vi "KE622x -- Set Arm Layer Params.vi"(0 "Resource In":refnum<visa-resource-name>, 1 "Check For SCPI Errors? (T)":bool=TRUE, 7 "Arm Layer Params In":T1={"Bypass Arm Layer\nInput Trigger?"=FALSE, "Input Trig Source"=enum."Immediate", "Input Trig Link Line"=enum."1", "Arm Timer Interval (s)"=0.001, "Output Trig Mode"=enum."No Trig Out", "Output Trig Link Line"=enum."1"} {"Arm Timer Interval (s)" min=0.001 max=99999.999 step=0.001 format="%.3f"}, 11 "error in (no error)":errorcluster, 12 "Read Back Set Values? (T)":bool=TRUE) -> (4 "Resource Out (dupl)":refnum<visa-resource-name>, 8 "Arm Layer Params Out":T1={"Bypass Arm Layer\nInput Trigger?"=FALSE, "Input Trig Source"=enum."Immediate", "Input Trig Link Line"=enum."1", "Arm Timer Interval (s)"=0.001, "Output Trig Mode"=enum."No Trig Out", "Output Trig Link Line"=enum."1"} {"Arm Timer Interval (s)" min=0.001 max=99999.999 step=0.001 format="%.3f"}, 15 "error out":errorcluster)   [LabVIEW 2019, in "Keithley 622x.lvlib"]
doc: "Sets the parameters for the 'Arm' layer of the trigger model."
uses:
  Keithley 622x.lvlib
  Typedefs/KE622x -- Arm Layer Params.ctl
  Low Level/Typedefs/KE622x -- Arm Source.ctl
  Low Level/Typedefs/KE622x -- Trig Link Line.ctl
  Low Level/Typedefs/KE622x -- Arm Timer Interval.ctl
  Low Level/Typedefs/KE622x -- Arm Output Mode.ctl
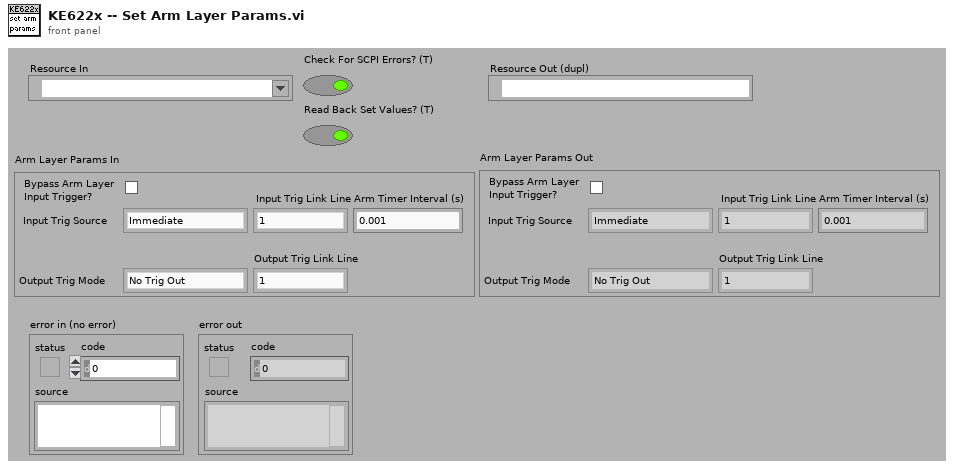
[diagram p1: front panel]
types:
  T1 = typedef "Keithley 622x.lvlib/KE622x -- Arm Layer Params.ctl" = cluster{"Bypass Arm Layer\nInput Trigger?":bool, "Input Trig Source":T2, "Input Trig Link Line":T3, "Arm Timer Interval (s)":T4, "Output Trig Mode":T5, "Output Trig Link Line":T3}
  T2 = typedef "Keithley 622x.lvlib/KE622x -- Arm Source.ctl" = enum16{"Immediate", "Bus (*TRG)", "Timer", "Manual", "Trigger Link", "SOT Falling Edge", "SOT Rising Edge", "SOT Either Edge"}
  T3 = typedef "Keithley 622x.lvlib/KE622x -- Trig Link Line.ctl" = enum16{"1", "2", "3", "4", "5", "6"}
  T4 = typedef "Keithley 622x.lvlib/KE622x -- Arm Timer Interval.ctl" = dbl
  T5 = typedef "Keithley 622x.lvlib/KE622x -- Arm Output Mode.ctl" = enum16{"No Trig Out", "Trig Out On Enter Arm", "Trig Out On Exit Arm"}
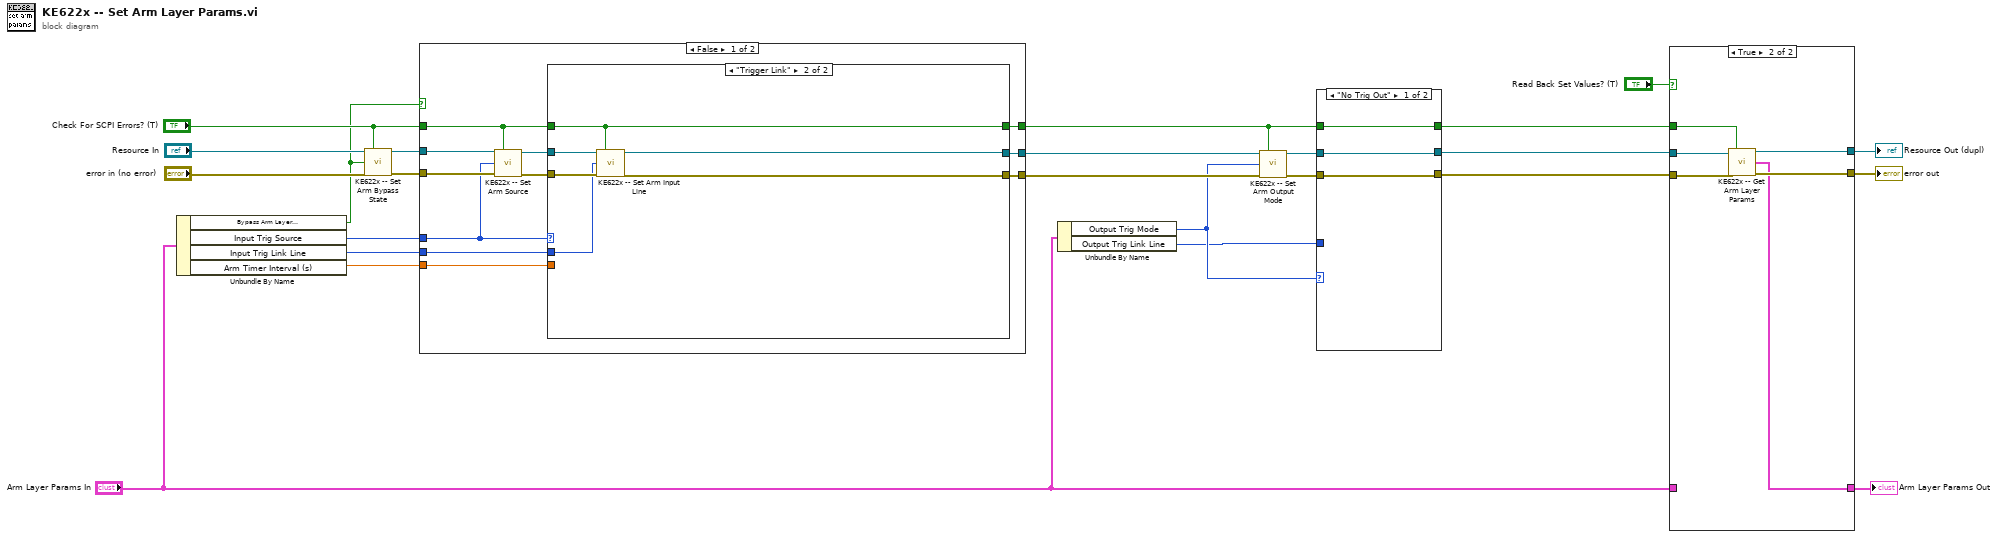
[diagram p0: block diagram]
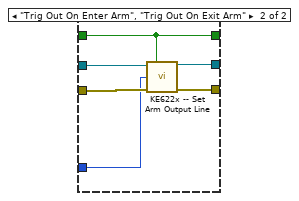
[diagram p2: hidden frame]
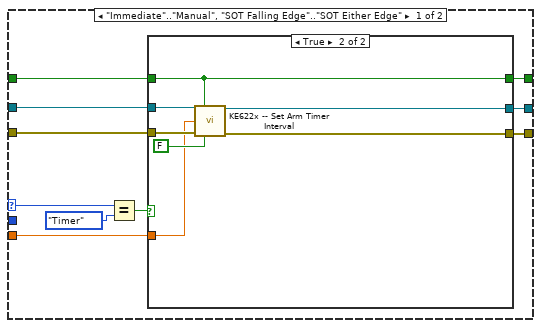
[diagram p3: hidden frame]
diagram:
  n1 = Unbundle By Name("Arm Layer Params In") -> ("Bypass Arm Layer\nInput Trigger?"=w16:bool, "Input Trig Source"=w15:T2, "Input Trig Link Line"=w14:T3, "Arm Timer Interval (s)"=w13:T4)
  n2 = call "KE622x -- Set Arm Bypass State.vi"("Resource In"="Resource In", "Check For SCPI Errors? (T)"="Check For SCPI Errors? (T)", "Bypass Arm Layer?"=w16, "error in (no error)"="error in (no error)") -> ("Resource Out (dupl)"=w23:refnum<visa-resource-name>, "error out"=w24:errorcluster)  [unwired: 10 in]
  n3 = case shown="False" w16 {
    tunnel: w24 -> [w35 w62]
    tunnel: w23 -> [w34 w63]
    tunnel: "Check For SCPI Errors? (T)" -> [w28 w64]
    tunnel: w15 -> [w33 _]
    tunnel: w14 -> [w32 _]
    tunnel: w13 -> [w31 _]
    tunnel: [w27 w63] -> w8
    tunnel: [w26 w62] -> w10
    tunnel: [w25 w64] -> w7
    frame False {
      n4 = call "KE622x -- Set Arm Source.vi"("Resource In"=w34, "Check For SCPI Errors? (T)"=w28, "Arm Source"=w33, "error in (no error)"=w35) -> ("Resource Out (dupl)"=w30:refnum<visa-resource-name>, "error out"=w29:errorcluster)  [unwired: 10 in]
      n5 = case shown="\"Trigger Link\"" w33 {
        selector: w33 -> [w45 _]
        tunnel: w32 -> [_ w59]
        tunnel: w31 -> [w39 _]
        tunnel: w30 -> [w42 w61]
        tunnel: w29 -> [w41 w60]
        tunnel: w28 -> [w40 w58]
        tunnel: [w38 w57] -> w27
        tunnel: [w37 w56] -> w26
        tunnel: [w36 w58] -> w25
        frame "Immediate".."Manual", "SOT Falling Edge".."SOT Either Edge" {
          n6 = Equal?(x=w45, y=KE622x_--_Arm_Source."Timer") -> (x = y?=w43:bool)
          n7 = case shown="True" w43 {
            tunnel: w42 -> [w48 w55]
            tunnel: w41 -> [w47 w54]
            tunnel: w40 -> [w46 w49]
            tunnel: w39 -> [_ w52]
            tunnel: [w48 w51] -> w38
            tunnel: [w47 w50] -> w37
            tunnel: [w46 w49] -> w36
            frame False {
            }
            frame True {
              n8 = call "KE622x -- Set Arm Timer Interval.vi"("Resource In"=w55, "Check For SCPI Errors? (T)"=w49, "Arm Timer Interval (s)"=w52, "error in (no error)"=w54, "Read Back Set Value? (T)"=FALSE) -> ("Resource Out (dupl)"=w51:refnum<visa-resource-name>, "error out"=w50:errorcluster)  [unwired: 8 in, 1 out]
            }
          }
        }
        frame "Trigger Link" {
          n9 = call "KE622x -- Set Arm Input Line.vi"("Resource In"=w61, "Check For SCPI Errors? (T)"=w58, "Arm Input Line"=w59, "error in (no error)"=w60) -> ("Resource Out (dupl)"=w57:refnum<visa-resource-name>, "error out"=w56:errorcluster)  [unwired: 10 in]
        }
      }
    }
    frame True {
    }
  }
  n10 = Unbundle By Name("Arm Layer Params In") -> ("Output Trig Mode"=w6:T5, "Output Trig Link Line"=w4:T3)
  n11 = call "KE622x -- Set Arm Output Mode.vi"("Resource In"=w8, "Check For SCPI Errors? (T)"=w7, "Arm Output Mode"=w6, "error in (no error)"=w10) -> ("Resource Out (dupl)"=w5:refnum<visa-resource-name>, "error out"=w9:errorcluster)  [unwired: 10 in]
  n12 = case shown="\"No Trig Out\"" w6 {
    tunnel: [w65 w73] -> w1
    tunnel: [w66 w72] -> w3
    tunnel: w9 -> [w65 w71]
    tunnel: w7 -> [w67 w68]
    tunnel: w5 -> [w66 w70]
    tunnel: w4 -> [_ w69]
    tunnel: [w67 w68] -> w2
    frame "No Trig Out" {
    }
    frame "Trig Out On Enter Arm", "Trig Out On Exit Arm" {
      n13 = call "KE622x -- Set Arm Output Line.vi"("Resource In"=w70, "Check For SCPI Errors? (T)"=w68, "Arm Output Line"=w69, "error in (no error)"=w71) -> ("Resource Out (dupl)"=w72:refnum<visa-resource-name>, "error out"=w73:errorcluster)  [unwired: 10 in]
    }
  }
  n14 = case shown="True" "Read Back Set Values? (T)" {
    tunnel: [w75 w82] -> w20
    tunnel: [w76 w81] -> w21
    tunnel: w3 -> [w76 w80]
    tunnel: w1 -> [w75 w79]
    tunnel: w2 -> [_ w78]
    tunnel: "Arm Layer Params In" -> [w74 _]
    tunnel: [w74 w77] -> w12
    frame False {
    }
    frame True {
      n15 = call "KE622x -- Get Arm Layer Params.vi"("Resource In"=w80, "Check For SCPI Errors? (T)"=w78, "error in (no error)"=w79) -> ("Resource Out (dupl)"=w81:refnum<visa-resource-name>, "Arm Params"=w77:T1, "error out"=w82:errorcluster)  [unwired: 10 in]
    }
  }
  "Resource Out (dupl)" <- w21
  "error out" <- w20
  "Arm Layer Params Out" <- w12
